vi "Handle Button Press.vi"(8 "error in (no error)":errorcluster, 10 "CtlRef":refnum<vi>, 11 "OneButtonDialogBox In":refnum<class "TwoButtonDialogBox.lvclass">) -> (0 "error out":errorcluster, 3 "OneButtonDialogBox Out":refnum<class "TwoButtonDialogBox.lvclass">)   [LabVIEW 2015, in "TwoButtonDialogBox.lvlib" / "TwoButtonDialogBox.lvclass"]
uses:
  TwoButtonDialogBox.lvclass
  <vilib>/ActorFramework/Actor/Actor.lvclass/Actor.ctl
  <vilib>/ActorFramework/Message Enqueuer/Message Enqueuer.lvclass/Message Enqueuer.ctl
  TwoButtonDialogBox.lvclass/TwoButtonDialogBox.ctl
  <vilib>/ActorFramework/Message Enqueuer/Init from Existing Queue.vi
  <vilib>/ActorFramework/Message Enqueuer/Enqueue.vi
  <vilib>/ActorFramework/Message Priority Queue/Priority Enqueue.vi
  <vilib>/ActorFramework/Message Enqueuer/Message Enqueuer.lvclass
  IDialogBox/IDialogBox Abstract Messages/Abstract Dialog Return Msg/Abstract Dialog Return Msg.lvclass
  <vilib>/ActorFramework/Stop Msg/Stop Msg.lvclass
  <vilib>/ActorFramework/Actor/Actor.lvclass
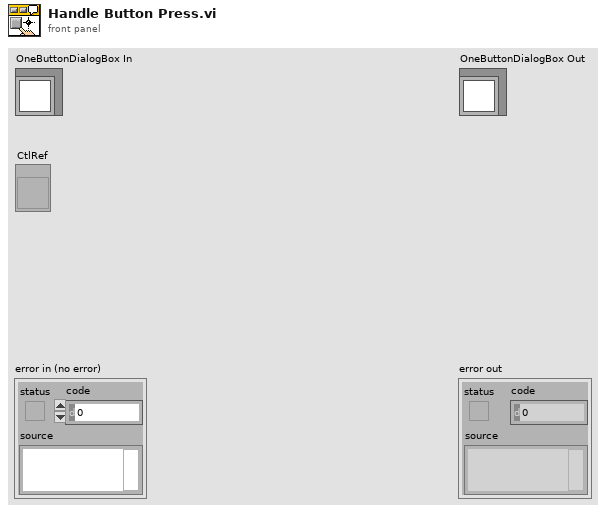
[diagram p1: front panel]
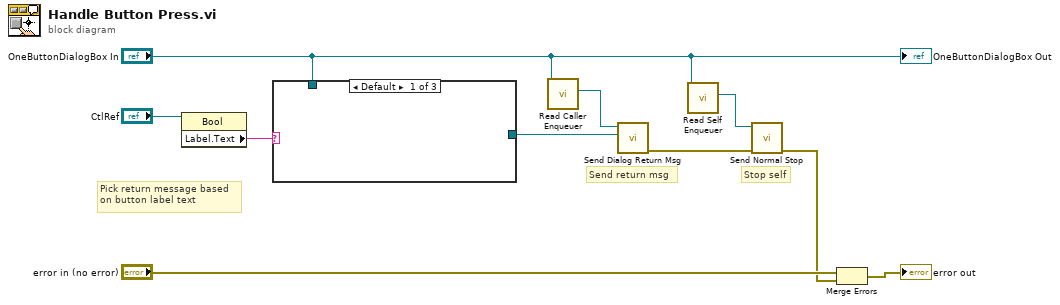
[diagram p0: block diagram]
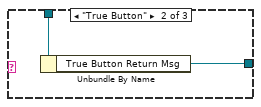
[diagram p2: hidden frame]
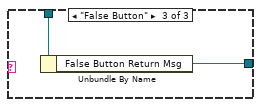
[diagram p3: hidden frame]
diagram:
  # "Pick return message based\non button label text"
  # "Stop self"
  # "Send return msg"
  n1 = property class="Bool"(reference="CtlRef") -> ("Label.Text"=w1:string)  [unwired: 1 in, 2 out]
  n2 = case shown="Default" w1 {
    tunnel: [_ w12 w14] -> w9
    tunnel: "OneButtonDialogBox In" -> [_ w11 w13]
    frame Default {
    }
    frame "True Button" {
      n3 = Unbundle By Name(w11) -> ("True Button Return Msg"=w12:refnum<class "Abstract Dialog Return Msg.lvclass">)
    }
    frame "False Button" {
      n4 = Unbundle By Name(w13) -> ("False Button Return Msg"=w14:refnum<class "Abstract Dialog Return Msg.lvclass">)
    }
  }
  n5 = call <vilib>:"Read Caller Enqueuer.vi"("Actor"="OneButtonDialogBox In") -> ("Caller Enqueuer"=w8:refnum<class "Message Enqueuer.lvclass">)  [unwired: 10 in]
  n6 = call "Send Dialog Return Msg.vi"("Dialog Return Msg"=w9, "Message Enqueuer in"=w8) -> ("error out"=w5:errorcluster)  [unwired: 9 in]
  n7 = call <vilib>:"Read Self Enqueuer.vi"("Actor"="OneButtonDialogBox In") -> ("Self Enqueuer"=w6:refnum<class "Message Enqueuer.lvclass">)  [unwired: 10 in]
  n8 = call <vilib>:"Send Normal Stop.vi"("error in (no error)"=w5, "Message Enqueuer"=w6) -> ("error out"=w3:errorcluster)  [unwired: 9 in]
  n9 = Merge Errors("error in (no error)", w3) -> (→"error out":errorcluster)
  "OneButtonDialogBox Out" <- "OneButtonDialogBox In"
